vi "Read Cycle time.vi"(8 "error in (no error)":errorcluster, 11 "BiStableShutter in":refnum<class "BiStableShutter.lvclass">) -> (0 "error out":errorcluster, 2 "Cycle time":dbl, 3 "BiStableShutter out":refnum<class "BiStableShutter.lvclass">)   [LabVIEW 2016, in "BiStableShutter.lvclass"]
uses:
  BiStableShutter.lvclass
  BiStableShutter.lvclass/BiStableShutter.ctl
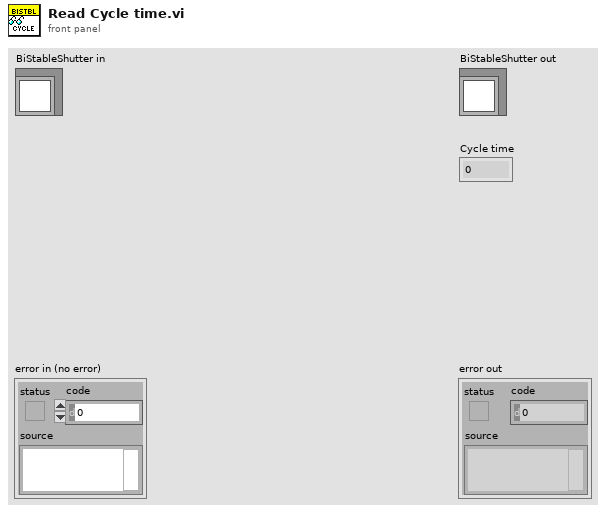
[diagram p1: front panel]
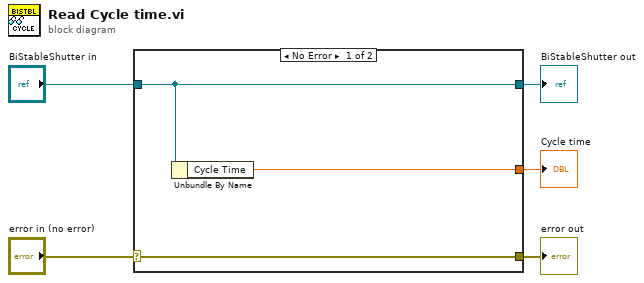
[diagram p0: block diagram]
diagram:
  n1 = case shown="No Error" "error in (no error)" {
    selector: "error in (no error)" -> [w8 w9]
    tunnel: [w8 w9] -> w4
    tunnel: [w7 w10] -> w2
    tunnel: "BiStableShutter in" -> [w7 w10]
    tunnel: [w6 _] -> w1
    frame No Error {
      n2 = Unbundle By Name(w7) -> ("Cycle Time"=w6:dbl)
    }
    frame Error {
    }
  }
  "error out" <- w4
  "BiStableShutter out" <- w2
  "Cycle time" <- w1
